vi "Convert_distance_to_command.vi"(11 "relative count":i32) -> (3 "command":string[](array[string]))   [LabVIEW 2017]
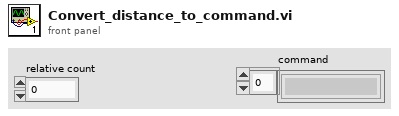
[diagram p1: front panel]
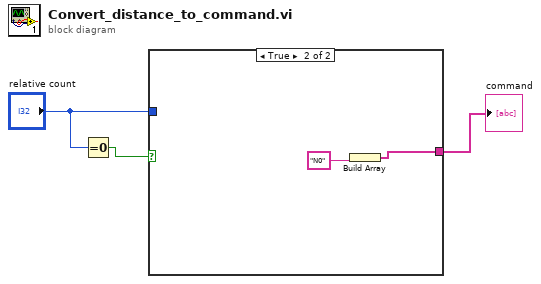
[diagram p0: block diagram]
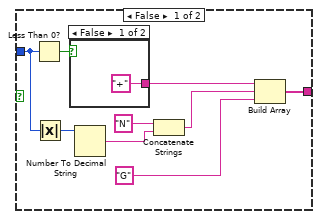
[diagram p2: hidden frame]
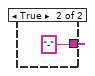
[diagram p3: hidden frame]
diagram:
  n1 = Equal To 0?(x="relative count") -> (x = 0?=w1:bool)
  n2 = case shown="TRUE" w1 {
    tunnel: "relative count" -> [w8 _]
    tunnel: [w4 w15] -> w3
    frame False {
      n3 = Less Than 0?(x=w8) -> (x < 0?=w11:bool)
      n4 = Absolute Value(x=w8) -> (abs(x)=w12:i32)
      n5 = case shown="FALSE" w11 {
        tunnel: ["+" "-"] -> w7
        frame False {
        }
        frame True {
        }
      }
      n6 = Number To Decimal String(number=w12) -> (decimal integer string=w10:string)  [unwired: 1 in]
      n7 = Concatenate Strings("N", w10) -> (w6:string)
      n8 = Build Array(w7, w6, "G") -> (w4:string[])
    }
    frame True {
      n9 = Build Array("N0") -> (w15:string[])
    }
  }
  "command" <- w3
